vi "Write Data.vi"(8 "error in (no error)":errorcluster, 10 "Base Data Lib:Data":refnum<class "Data.lvclass">, 11 "Send Data to Caller in":refnum<class "Send Data to Caller.lvclass">) -> (0 "error out":errorcluster, 3 "Send Data to Caller out":refnum<class "Send Data to Caller.lvclass">)   [LabVIEW 2014, in "Send Data to Caller.lvclass"]
uses:
  Send Data to Caller.lvclass
  Data/Data.lvclass
  Send Data to Caller.lvclass/Send Data to Caller.ctl
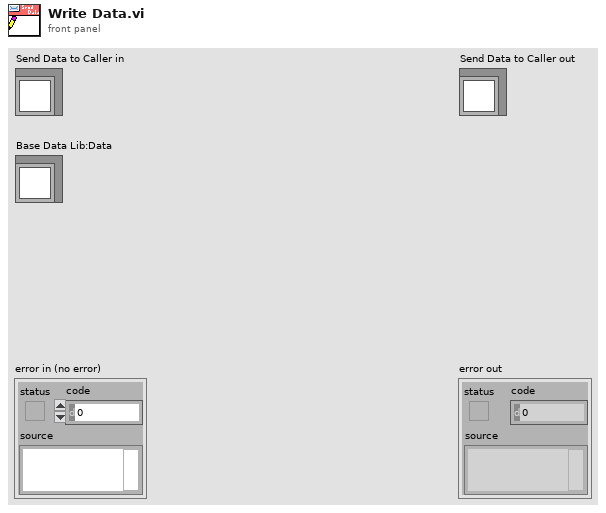
[diagram p1: front panel]
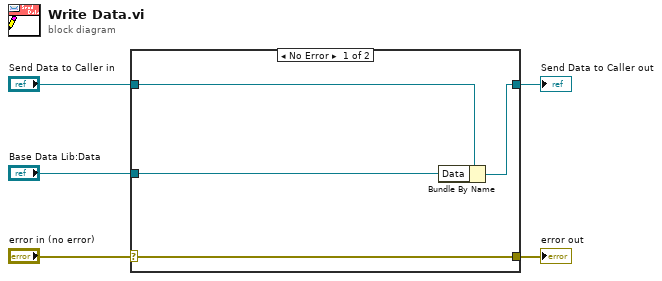
[diagram p0: block diagram]
diagram:
  n1 = case shown="No Error" "error in (no error)" {
    selector: "error in (no error)" -> [w9 w10]
    tunnel: [w9 w10] -> w4
    tunnel: [w7 w11] -> w2
    tunnel: "Send Data to Caller in" -> [w8 w11]
    tunnel: "Base Data Lib:Data" -> [w6 _]
    frame No Error {
      n2 = Bundle By Name(cluster=w8, "Data"=w6) -> (w7:refnum<class "Send Data to Caller.lvclass">)
    }
    frame Error {
    }
  }
  "error out" <- w4
  "Send Data to Caller out" <- w2
